vi "RT Driver VI.vi"(7 "Operation":T1, 11 "Device Reference in":T2 format="%.0x") -> (0 "Error Code":i32)   [LabVIEW 2019, in "Profile Interpolation Engine.lvlib"]
uses:
  Profile Interpolation Engine.lvlib
  <vilib>/NI VeriStand/Custom Device API/Custom Device Item Ref.ctl
  <vilib>/NI VeriStand/Custom Device API/Hardware Interface Driver VI Operation.ctl
  Shared/Types/Compiled.Settings.ctl
  <vilib>/NI VeriStand/Custom Device API/Custom Device Target Type.ctl
  Types/RTStateVariables.ctl
  <vilib>/NI/NIVS Inline Async API/_VS Inline Async API/VS Inline Async API/VS Inline Async API.lvclass
  <vilib>/NI/NIVS Inline Async API/_VS Inline Async API/VS Inline Async API/VS Inline Async API.lvclass/VS Inline Async API.ctl
  <vilib>/NI/NIVS Inline Async API/_Data Access Engine/Data Access Engine/Data Access Engine.lvclass/Data Access Engine.ctl
  <vilib>/NI/NIVS Inline Async API/_Data Access Engine/Access Type Classes/Write/Write.lvclass/Write.ctl
  <vilib>/NI/NIVS Inline Async API/_Data Access Engine/Access Type Classes/ReadWrite/ReadWrite.lvclass/ReadWrite.ctl
  <vilib>/NI/NIVS Inline Async API/_Data Access Engine/Access Type Classes/Read/Read.lvclass/Read.ctl
  <vilib>/NI/NIVS Inline Async API/_Data Access Engine/Data Access Engine/Methods/Data.Engine.Read Data from HW.vi
  <vilib>/NI/NIVS Inline Async API/_VS Inline Async API/Error Handling Process/SubVIs/Error.GetError.vi
  <vilib>/NI/NIVS Inline Async API/_Data Access Engine/Data Access Engine/Methods/Data.Engine.Write Data to HW.vi
  <vilib>/NI/NIVS Inline Async API/_Data Access Engine/Access Type Classes/ReadWrite/ReadWrite.EngineData.vi
  <vilib>/NI/NIVS Inline Async API/_Data Access Engine/Access Type Classes/Write/Write.EngineData.vi
  <vilib>/NI/NIVS Inline Async API/_Data Access Engine/Access Type Classes/Read/Read.EngineData.vi
  <vilib>/NI VeriStand/Custom Device API/NI VeriStand - Get Channel Value by Data Reference.vi
  <vilib>/NI VeriStand/Custom Device API/NI VeriStand - Set Channel Value by Data Reference.vi
  <vilib>/NI VeriStand/Custom Device API/NI VeriStand - Get Channel Values by Block Data Reference.vi
  Shared/SubVIs/Constants.vi
  <vilib>/NI VeriStand/Custom Device API/Get Item Property (Variant).vi
  <vilib>/NI VeriStand/Custom Device API/Get Item Property (Dependent File).vi
  <vilib>/NI VeriStand/Custom Device Tools/Custom Device Utility Library/NI VeriStand - Search for Item by GUID.vi
  <userlib>/_OpenG.lib/array/array.llb/Sort 1D Array (String)__ogtk.vi
  Profile Interpolation Custom Device.Async.vi
  <vilib>/NI VeriStand/Custom Device API/Global Data Refs.vi
  <vilib>/NI VeriStand/Custom Device API/Custom Device API.lvlib
  <vilib>/NI VeriStand/Custom Device Tools/Custom Device Utility Library/Custom Device Utility Library.lvlib
  Shared/Profile Interpolation Shared.lvlib
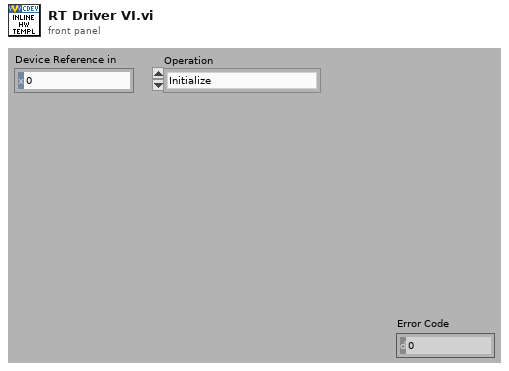
[diagram p1: front panel]
types:
  T1 = typedef "Custom Device API.lvlib/Hardware Interface Driver VI Operation.ctl" = enum16{"Initialize", "Start", "Read Data from HW", "Write Data to HW", "Close"}
  T2 = typedef "Custom Device API.lvlib/Custom Device Item Ref.ctl" = u64
  T3 = typedef "Profile Interpolation Engine.lvlib/RTStateVariables.ctl" = cluster{"Async":refnum<class "VS Inline Async API.lvclass">, "Settings":T4}
  T4 = typedef "Profile Interpolation Shared.lvlib/Compiled.Settings.ctl" = cluster{"Name":string, "Create Limit Channels?":bool, "Profiles []":cluster{"Profile":dbl[][]}[], "Target.Type":T5}
  T5 = typedef "Custom Device API.lvlib/Custom Device Target Type.ctl" = enum16{"PharLap", "VxWorks", "Windows", "Linux_32_ARM", "Linux_x64"}
  T6 = typedef "Custom Device API.lvlib/Dependent File Optional Info.ctl" = cluster{"Version":string, "RTDestination":path, "ForceDownload":bool, "SupportedTarget":string, "MD5":string}
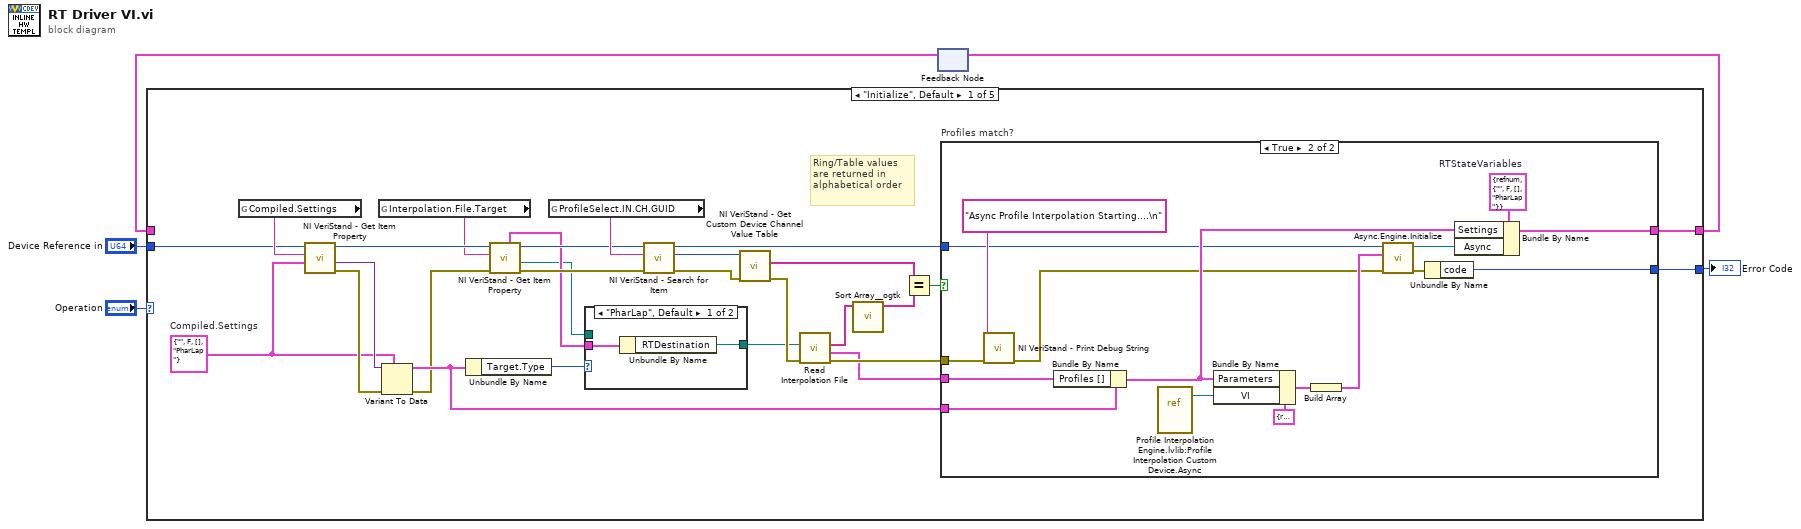
[diagram p0: block diagram]
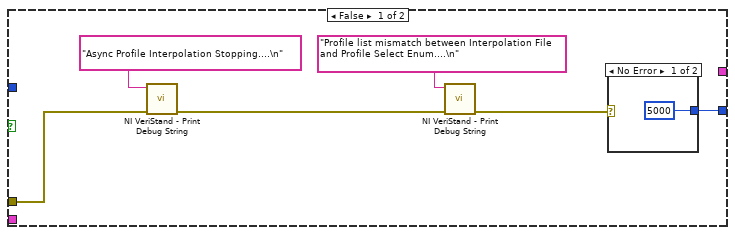
[diagram p3: hidden frame]
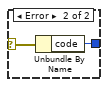
[diagram p4: hidden frame]
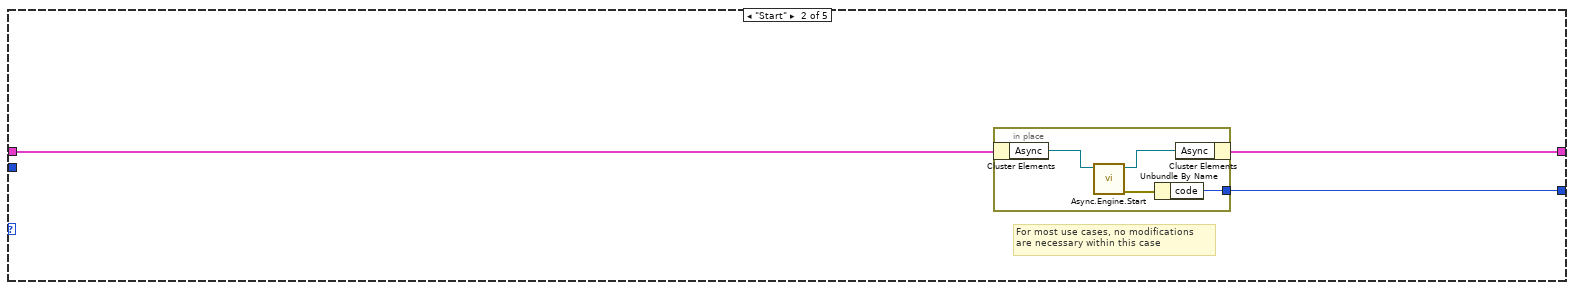
[diagram p5: hidden frame]
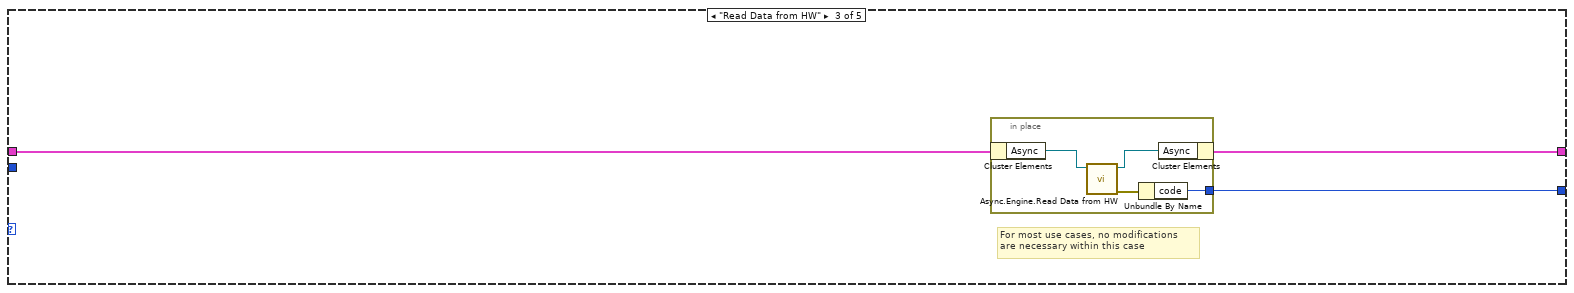
[diagram p6: hidden frame]
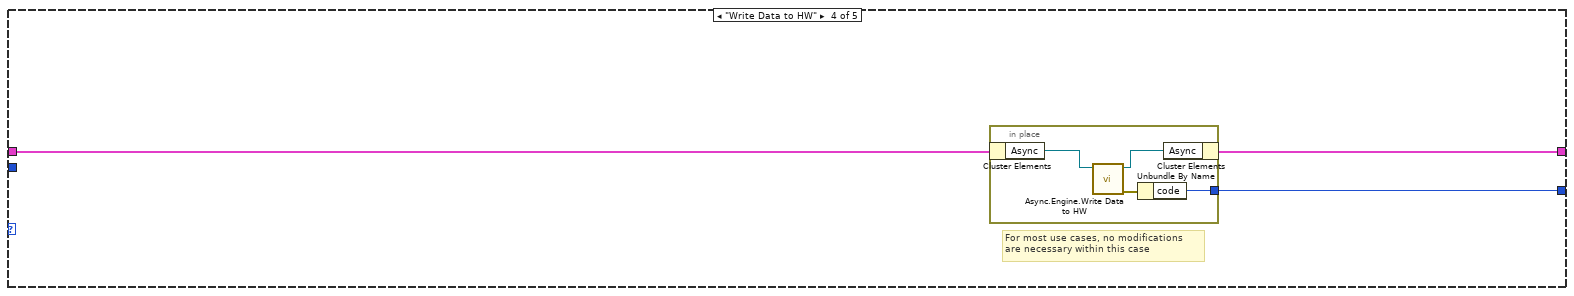
[diagram p7: hidden frame]
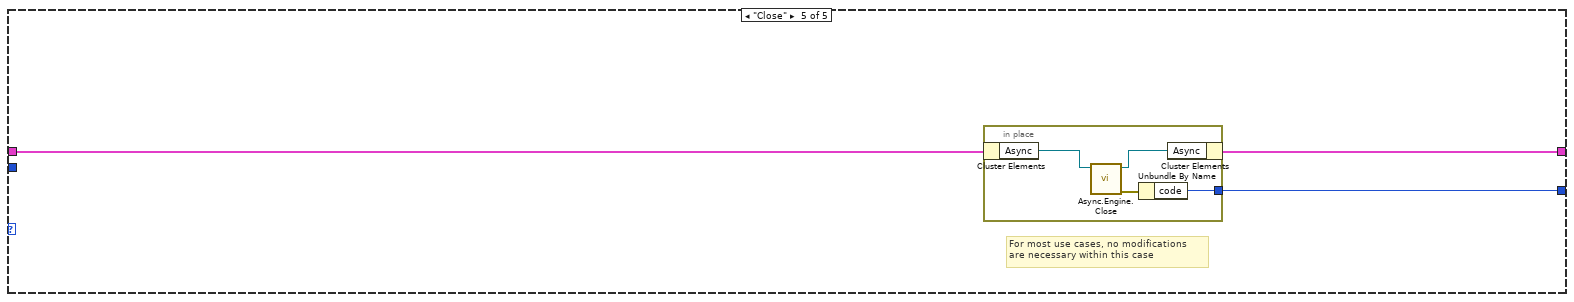
[diagram p8: hidden frame]
diagram:
  n1 = feedback #1() -> (w3:T3)  [unwired: 1 out]
  n2 = case shown="\"Initialize\", Default" "Operation" {
    tunnel: [w32 w63 w69 w76 w84] -> w4
    tunnel: w3 -> [_ w64 w71 w77 w85]
    tunnel: "Device Reference in" -> [w19 _ _ _ _]
    tunnel: [w33 w62 w70 w78 w83] -> w1
    frame "Initialize", Default {
      w20 = T4 {"Name"="", "Create Limit Channels?"=FALSE, "Profiles []"=[], "Target.Type"=enum."PharLap"}  # Compiled.Settings
      # "Ring/Table values are returned in alphabetical order"
      n3 = global read "Constants.vi" "Compiled.Settings"() -> (w21:string)
      n4 = call-poly <vilib>:"NI VeriStand - Get Item Property.vi"("Default Value"=w20, "Property Name"=w21, "Item Ref in"=w19) -> ("error out"=w23:errorcluster, "Value"=w22:variant, "Item Ref out"=w16:T2)  [unwired: 5 in, 1 out]
      n5 = global read "Constants.vi" "Interpolation.File.Target"() -> (w11:string)
      n6 = Variant To Data(error in=w23, type=w20, Variant=w22) -> (data=w18:T4, error out=w17:errorcluster)
      n7 = Unbundle By Name(w18) -> ("Target.Type"=w13:T5)
      n8 = call-poly <vilib>:"NI VeriStand - Get Item Property.vi"("error in (no error)"=w17, "Property Name"=w11, "Item Ref in"=w16) -> ("error out"=w14:errorcluster, "Path"=w9:path, "Item Ref out"=w15:T2, "OptionalInfo"=w10:T6)  [unwired: 4 in, 1 out]
      n9 = global read "Constants.vi" "ProfileSelect.IN.CH.GUID"() -> (w28:string)
      n10 = case shown="\"PharLap\", Default" w13 {
        tunnel: w9 -> [_ w36]
        tunnel: [w34 w36] -> w12
        tunnel: w10 -> [w35 _]
        frame "PharLap", Default {
          n11 = Unbundle By Name(w35) -> ("RTDestination"=w34:path)
        }
        frame "Windows" {
        }
      }
      n12 = call-poly <vilib>:"NI VeriStand - Search for Item.vi"("error in"=w14, "Item GUID"=w28, "Section Ref in"=w15) -> ("error out"=w31:errorcluster, "Item Ref"=w30:T2, "Section Ref out"=w27:T2)  [unwired: 5 in, 1 out]
      n13 = call <vilib>:"NI VeriStand - Get Custom Device Channel Value Table.vi"("error in (no error)"=w31, "Channel Ref in"=w30) -> ("error out"=w29:errorcluster, "Names"=w8:string[])  [unwired: 6 in, 2 out]
      n14 = call "Read Interpolation File.vi"("error in"=w29, "file path (dialog if empty)"=w12) -> ("error out"=w26:errorcluster, "Profiles []"=w24:cluster{"Profile":dbl[][]}[], "Profiles"=w7:string[])  [unwired: 2 in, 5 out]
      n15 = call-poly <userlib>:"Sort Array__ogtk.vi"("Array in"=w7) -> ("Sorted Array out"=w6:string[])  [unwired: 9 in, 1 out]
      n16 = Equal?(x=w8, y=w6) -> (x = y?=w25:bool)
      n17 = case "Profiles match?" shown="True" w25 {
        tunnel: [w42 w61] -> w33
        tunnel: [_ w59] -> w32
        tunnel: w27 -> [_ w48]
        tunnel: w26 -> [w41 w51]
        tunnel: w24 -> [_ w49]
        tunnel: w18 -> [_ w46]
        frame False {
          n18 = call <vilib>:"NI VeriStand - Print Debug String.vi"("error in (no error)"=w41, "Message"="Async Profile Interpolation Stopping....\n") -> ("error out"=w38:errorcluster)  [unwired: 9 in]
          n19 = call <vilib>:"NI VeriStand - Print Debug String.vi"("error in (no error)"=w38, "Message"="Profile list mismatch between Interpolation File and Profile Select Enum....\n") -> ("error out"=w37:errorcluster)  [unwired: 9 in]
          n20 = case shown="No Error" w37 {
            selector: w37 -> [_ w44]
            tunnel: [5000 w45] -> w42
            frame No Error {
            }
            frame Error {
              n21 = Unbundle By Name(w44) -> ("code"=w45:i32)
            }
          }
        }
        frame True {
          w55 = T3 {"Async"=refnum, "Settings"={"Name"="", "Create Limit Channels?"=FALSE, "Profiles []"=[], "Target.Type"=enum."PharLap"}}  # RTStateVariables
          n22 = call <vilib>:"NI VeriStand - Print Debug String.vi"("error in (no error)"=w51, "Message"="Async Profile Interpolation Starting....\n") -> ("error out"=w47:errorcluster)  [unwired: 9 in]
          n23 = Bundle By Name(cluster=w46, "Profiles []"=w49) -> (w50:T4)
          n24 = vi-ref "Profile Interpolation Engine.lvlib:Profile Interpolation Custom Device.Async.vi"() -> (w52:refnum<vi>)
          n25 = Bundle By Name(cluster=cluster{"VI":refnum<vi>, "Parameters":variant} {"VI"=refnum, "Parameters"=variant} ("Process"), "Parameters"=w50, "VI"=w52) -> (w57:cluster{"VI":refnum<vi>, "Parameters":variant})
          n26 = Build Array(w57) -> (w54:cluster{"VI":refnum<vi>, "Parameters":variant}[])
          n27 = call <vilib>:"Async.Engine.Initialize.vi"("error in (no error)"=w47, "Processes"=w54, "Custom Device Ref"=w48) -> ("error out"=w56:errorcluster, "Async"=w60:refnum<class "VS Inline Async API.lvclass">)  [unwired: 7 in]
          n28 = Unbundle By Name(w56) -> ("code"=w61:i32)
          n29 = Bundle By Name(cluster=w55, "Settings"=w50, "Async"=w60) -> (w59:T3)
        }
      }
    }
    frame "Start" {
      # "For most use cases, no modifications \nare necessary within this case"
      n30 = in-place {
        in-place-border: [w65] -> w62
        n31 = in-place-cluster #2(w64) -> ("Async"=w68:refnum<class "VS Inline Async API.lvclass">)
        n32 = call <vilib>:"Async.Engine.Start.vi"("VS Inline Async API in"=w68) -> ("error out"=w66:errorcluster, "VS Inline Async API out"=w67:refnum<class "VS Inline Async API.lvclass">)  [unwired: 9 in]
        n33 = Unbundle By Name(w66) -> ("code"=w65:i32)
        n34 = in-place-cluster #2("Async"=w67) -> (w63:T3)
      }
    }
    frame "Read Data from HW" {
      # "For most use cases, no modifications \nare necessary within this case"
      n35 = in-place {
        in-place-border: [w73] -> w70
        n36 = in-place-cluster #3(w71) -> ("Async"=w75:refnum<class "VS Inline Async API.lvclass">)
        n37 = call <vilib>:"Async.Engine.Read Data from HW.vi"("Async in"=w75) -> ("error out"=w72:errorcluster, "Async out"=w74:refnum<class "VS Inline Async API.lvclass">)  [unwired: 9 in]
        n38 = Unbundle By Name(w72) -> ("code"=w73:i32)
        n39 = in-place-cluster #3("Async"=w74) -> (w69:T3)
      }
    }
    frame "Write Data to HW" {
      # "For most use cases, no modifications \nare necessary within this case"
      n40 = in-place {
        in-place-border: [w82] -> w78
        n41 = in-place-cluster #4(w77) -> ("Async"=w80:refnum<class "VS Inline Async API.lvclass">)
        n42 = call <vilib>:"Async.Engine.Write Data to HW.vi"("VS Inline Async API in"=w80) -> ("error out"=w81:errorcluster, "VS Inline Async API out"=w79:refnum<class "VS Inline Async API.lvclass">)  [unwired: 9 in]
        n43 = Unbundle By Name(w81) -> ("code"=w82:i32)
        n44 = in-place-cluster #4("Async"=w79) -> (w76:T3)
      }
    }
    frame "Close" {
      # "For most use cases, no modifications \nare necessary within this case"
      n45 = in-place {
        in-place-border: [w87] -> w83
        n46 = in-place-cluster #5(w85) -> ("Async"=w89:refnum<class "VS Inline Async API.lvclass">)
        n47 = call <vilib>:"Async.Engine.Close.vi"("Async in"=w89) -> ("error out"=w86:errorcluster, "Async out"=w88:refnum<class "VS Inline Async API.lvclass">)  [unwired: 9 in]
        n48 = Unbundle By Name(w86) -> ("code"=w87:i32)
        n49 = in-place-cluster #5("Async"=w88) -> (w84:T3)
      }
    }
  }
  "Error Code" <- w1
  n50 = feedback-in #1(w4) -> ()
